vi "GetMultipleFilesPath.vi"(10 "Path":path) -> (2 "PathArray":path[](array[path]))   [LabVIEW 2012]
panel:
  in  "Reload":bool
  in  "Start":bool
  in  "Selected Files#":i32[](listbox)
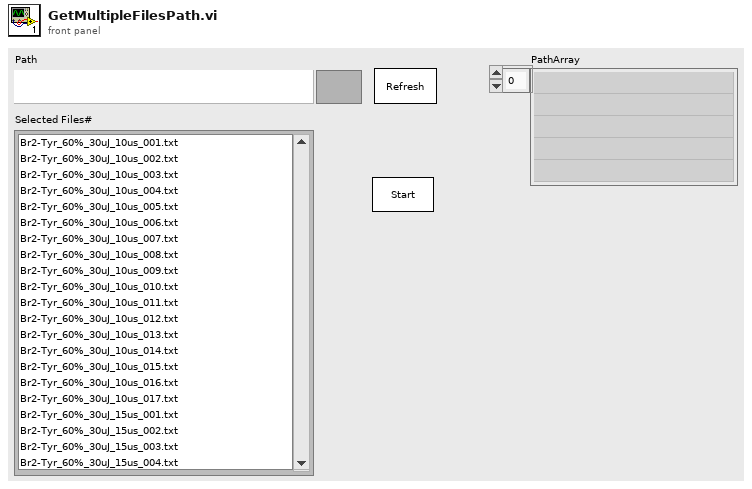
[diagram p1: front panel]
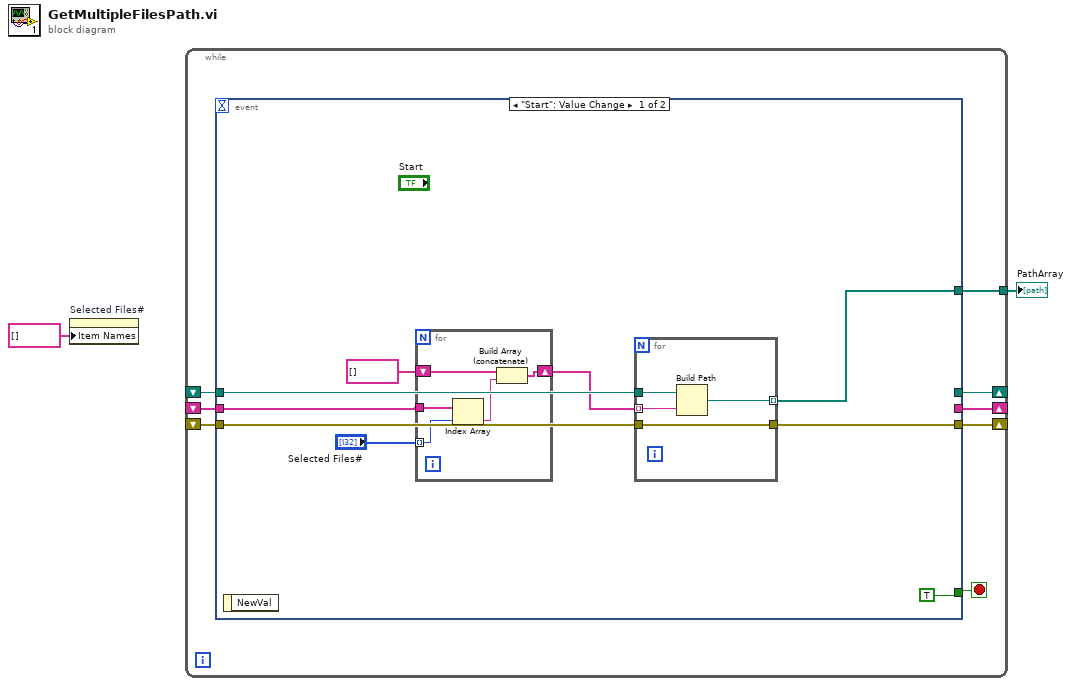
[diagram p0: block diagram]
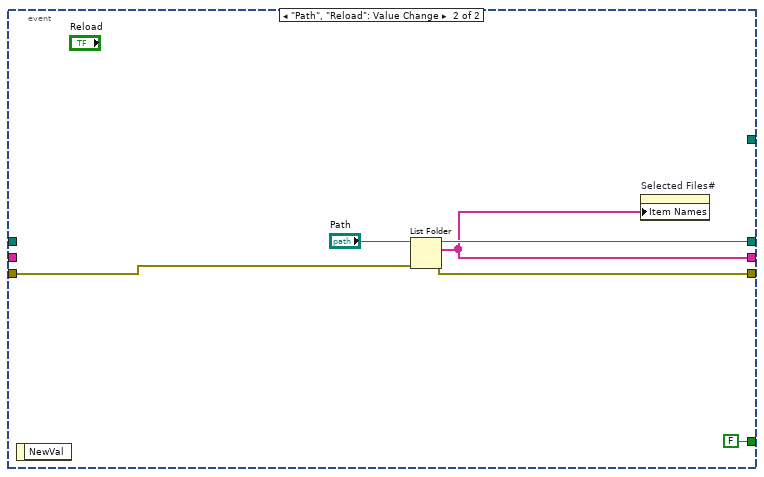
[diagram p2: hidden frame]
diagram:
  n1 = property on="Selected Files#" class="LstBox (strict)"("Item Names"=string[] []) -> ()  [unwired: 2 in, 2 out]
  n2 = while {
    shift-right: [w7] -> _
    shift-left: _ -> [w10]
    shift-right: [w8] -> _
    shift-left: _ -> [w9]
    shift-right: [w5] -> _
    shift-left: _ -> [w6]
    tunnel: [w3] -> w1
    stop <- w4 stop-if-true
    n3 = event shown="[0] \"Start\": Value Change" {
      selector: _ -> [_ _]
      dyn-events: _ -> [_ _]
      timeout: _ -> [_ _]
      tunnel: w10 -> [w13 _]
      tunnel: w9 -> [w19 w30]
      tunnel: [w18 w31] -> w8
      tunnel: [_ w32] -> w7
      tunnel: w6 -> [w17 _]
      tunnel: [_ w33] -> w5
      tunnel: [TRUE FALSE] -> w4
      tunnel: [w12 _] -> w3
      event "Start": Value Change {
        n4 = event-data() -> ()  [unwired: 1 in, 1 out]
        n5 = for {
          tunnel: "Selected Files#" -> [w21] mode=indexing
          tunnel: w13 -> [w22]
          shift-right: [w23] -> w14
          shift-left: string[] [] ("filenames") -> [w24]
          n6 = Index Array(array=w22, index=w21) -> (element=w20:string)
          n7 = Build Array (concatenate)(w24, w20) -> (w23:string[])
        }
        n8 = for {
          tunnel: w17 -> [w27]
          tunnel: w14 -> [w28] mode=indexing
          tunnel: w19 -> [w26]
          tunnel: [w26] -> w18
          tunnel: [w25] -> w12 mode=indexing
          n9 = Build Path(base path=w27, name or relative path=w28) -> (appended path=w25:path)
        }
      }
      event "Path", "Reload": Value Change {
        n10 = event-data() -> ()  [unwired: 1 in, 1 out]
        n11 = List Folder(path="Path", error in=w30) -> (path out=w33:path, filenames=w32:string[], error out=w31:errorcluster)  [unwired: 2 in, 1 out]
        n12 = property on="Selected Files#" class="LstBox (strict)"("Item Names"=w32) -> ()  [unwired: 2 in, 2 out]
      }
    }
  }
  "PathArray" <- w1
